vi "New TCP Socket Connection.vi"(8 "error in (no error)":errorcluster, 9 "timeout ms (5000)":i32=5000, 10 "Port":u16, 11 "Hostname / IP":string) -> (0 "error out":errorcluster, 3 "VISA TCP out":refnum<class "VISA TCP.lvclass">)   [LabVIEW 2021, in "Sockets.lvlib" / "VISA TCP.lvclass"]
doc: "Opens a new TCP Socket connection on the given hostname/port.\nWebSockets 2.0.1.40\nSam Sharp - MediaMongrels Ltd\nCopyright (c) 2019, MediaMongrels Ltd"
uses:
  VISA TCP.lvclass
  VISA TCP.lvclass/VISA TCP.ctl
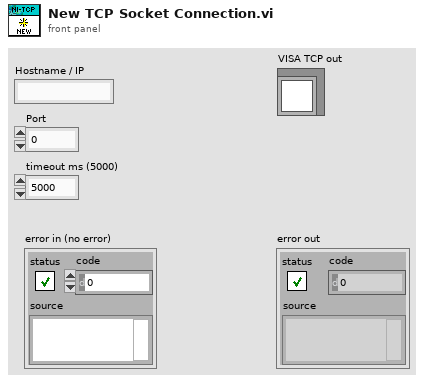
[diagram p1: front panel]
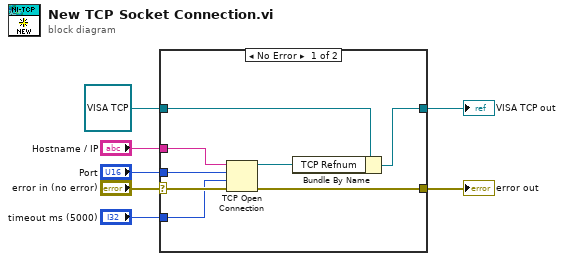
[diagram p0: block diagram]
diagram:
  n1 = case shown="No Error" "error in (no error)" {
    selector: "error in (no error)" -> [w11 w17]
    tunnel: [w12 w17] -> w6
    tunnel: [w14 w16] -> w5
    tunnel: refnum<class "VISA TCP.lvclass"> refnum ("VISA TCP in") -> [w15 w16]
    tunnel: "Hostname / IP" -> [w10 _]
    tunnel: "Port" -> [w9 _]
    tunnel: "timeout ms (5000)" -> [w8 _]
    frame No Error {
      n2 = TCP Open Connection(address=w10, remote port or service name=w9, timeout ms (60000)=w8, error in (no error)=w11) -> (connection ID=w13:refnum<k5>, error out=w12:errorcluster)  [unwired: 1 in]
      n3 = Bundle By Name(cluster=w15, "TCP Refnum"=w13) -> (w14:refnum<class "VISA TCP.lvclass">)
    }
    frame Error {
    }
  }
  "error out" <- w6
  "VISA TCP out" <- w5
